vi "Untitled 4.vi"() -> ()   [LabVIEW 2018]
uses:
  2D/IV/IV.lvclass
  2D/IV/meas/IV_meas.lvclass
panel:
  out "IV out":refnum<class "IV.lvclass">
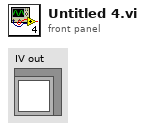
[diagram p1: front panel]
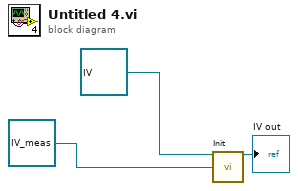
[diagram p0: block diagram]
diagram:
  n1 = call-dynamic "Init.vi"("IV in"=refnum<class "IV.lvclass"> refnum, "Measurement2D.lvclass"=refnum<class "IV_meas.lvclass"> refnum ("IV_meas.lvclass")) -> ("IV out"=→"IV out":refnum<class "IV.lvclass">)  [unwired: 12 in, 1 out]
